vi "svx_Colormap Frequency Area In.vi"(5 "Order":dbl, 7 "Range":T1, 11 "speed profile":cluster{"time [s]":dbl[], "speed [rpm]":dbl[]} {"speed [rpm]" format="%.2f"; "time [s]" format="%.2f"}) -> (0 "Order":dbl[](array[numeric]), 3 "Time(s)":dbl[](array[numeric]))   [LabVIEW 2017, in "SVX Colormap.xctl"]
uses:
  <vilib>/addons/_XControls/Colormap/SVX Colormap.xctl
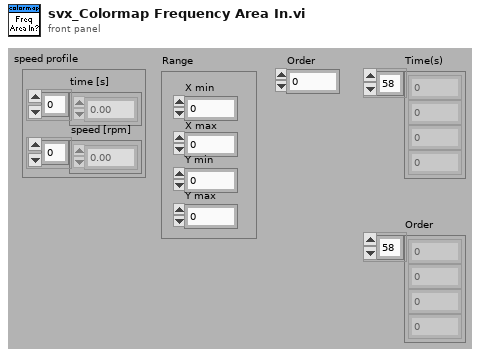
[diagram p1: front panel]
types:
  T1 = cluster{"X min":dbl, "X max":dbl, "Y min":dbl, "Y max":dbl}
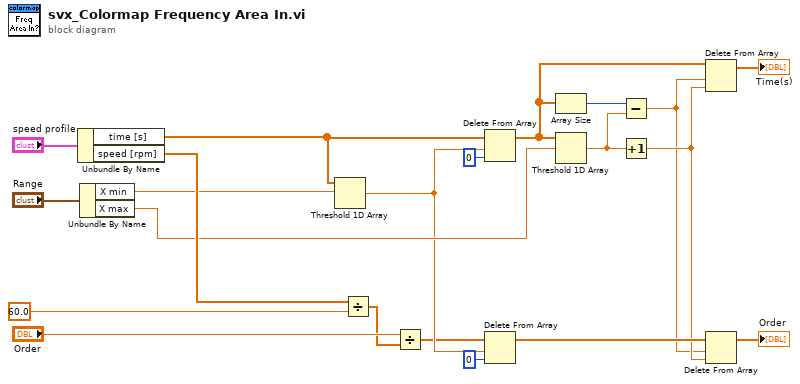
[diagram p0: block diagram]
diagram:
  n1 = Unbundle By Name("speed profile") -> ("time [s]"=w12:dbl[], "speed [rpm]"=w13:dbl[])
  n2 = Unbundle By Name("Range") -> ("X min"=w11:dbl, "X max"=w10:dbl)
  n3 = Threshold 1D Array(2:w11, 3:w12) -> (0:w9:dbl)  [unwired: 1 in]
  n4 = Divide(x=w13, y=60.0) -> (x/y=w1:dbl[])
  n5 = Divide(x="Order", y=w1) -> (x/y=w3:dbl[])
  n6 = Delete From Array(array=w12, length=w9, index=0) -> (array with subset deleted=w15:dbl[])  [unwired: 1 out]
  n7 = Delete From Array(array=w3, length=w9, index=0) -> (array with subset deleted=w17:dbl[])  [unwired: 1 out]
  n8 = Array Size(array=w15) -> (size(s)=w20:i32)
  n9 = Threshold 1D Array(2:w10, 3:w15) -> (0:w19:dbl)  [unwired: 1 in]
  n10 = Subtract(x=w20, y=w19) -> (x-y=w14:dbl)
  n11 = Increment(x=w19) -> (x+1=w16:dbl)
  n12 = Delete From Array(array=w15, length=w14, index=w16) -> (array with subset deleted=→"Time(s)":dbl[])  [unwired: 1 out]
  n13 = Delete From Array(array=w17, length=w14, index=w16) -> (array with subset deleted=→"Order":dbl[])  [unwired: 1 out]
